vi "sub_NtripClient_TCP.vi"(8 "error in":errorcluster) -> (0 "error out":errorcluster)   [LabVIEW 2019]
uses:
  Ctrl/comm-ini-rw-close.ctl
  Ctrl/cmd_common.ctl
  Ctrl/cmd_RW.ctl
  Ctrl/cmd_ini-RW.ctl
panel:
  out "n":i32
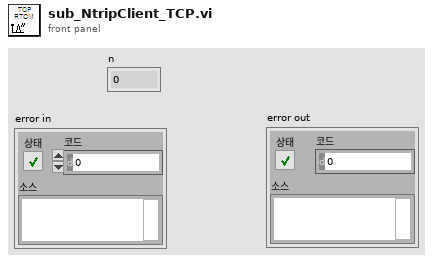
[diagram p1: front panel]
types:
  T1 = typedef "cmd_common.ctl" = enum16{"read", "write"}
  T2 = typedef "comm-ini-rw-close.ctl" = enum16{"ini", "write", "read", "close"}
  T3 = typedef "cmd_ini-RW.ctl" = enum16{"ini", "read", "write"}
  T4 = typedef "cmd_RW.ctl" = enum16{"read", "write"}
  T5 = typedef "GNSS-Ntrip config.ctl" = cluster{"Ntrip accounts DB":T6[], "Mount points":u16, "Ref r size":dbl, "TMarr limit":i32, "Sel NMEA type":enum16{"$GPGSV", "$GLGSV", "$GPGGA", "$GAGSV", "$GBGSV", "$GNGLL", "$GNGGA", "$GNGSA", "$GNRMC", "$GNVTG"}, "Local Time offset":u32, "GNSS Serial delay":u32, "Send Serial delay":u32, "Send Serial config":cluster{"NMEA out port":refnum<visa-resource-name>, "baud rate":u32}, "Mount point arr":string[], "Ntrip account DB index":u32}
  T6 = typedef "Ntrip_Account_db.ctl" = cluster{"address":string, "port ":u16, "id":string, "pwd":string, "ref pt":string}
  T7 = cluster{"Ntrip tcp":bool, "GNSS serial":bool, "RTCM serial":bool, "Send serial":bool}
  T8 = typedef "GNSS-Ntrip process val.ctl" = cluster{"GNSS time":string, "Ntrip conn":bool, "NMEA val":bool, "ycenter_TM":dbl, "xcenter_TM":dbl, "TM ref circles":cluster{"Y(E)":dbl, "X(N)":dbl}[], "RTCM recv-str":string, "GNSS Serail buff N":u32, "Sel NMEA type":enum16{"$GPGSV", "$GLGSV", "$GPGGA", "$GAGSV", "$GBGSV", "$GNGLL", "$GNGGA", "$GNGSA", "$GNRMC", "$GNVTG"}, "RTCM recv_sourcetable":string, "NMEA cluster":cluster{"GxGGA":string, "GxGSV":string, "GNRMC":string, "GxTXT":string, "GxGSA":string, "GxGLL":string}, "Sel NMEA str":string, "NMEA recv-str":string}
  T9 = typedef "GNSS-Ntrip ref.ctl" = cluster{"Mount point arr":refnum<vi>, "Select Mount points":refnum<vi>}
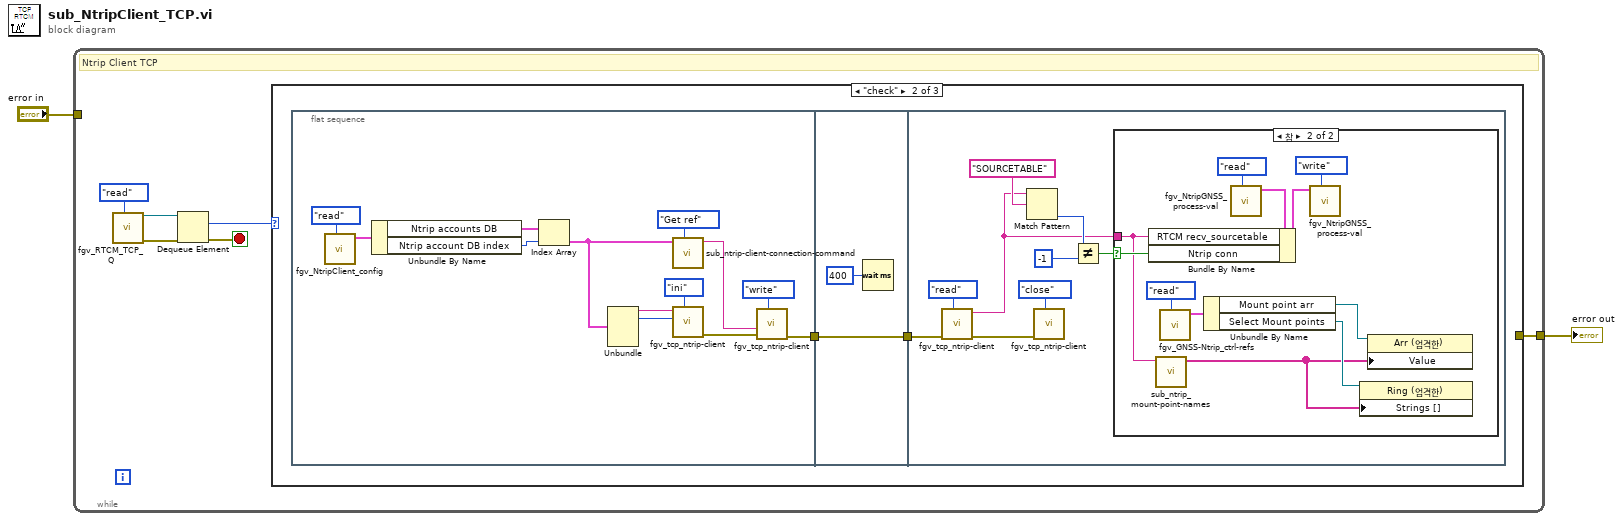
[diagram p0: block diagram]
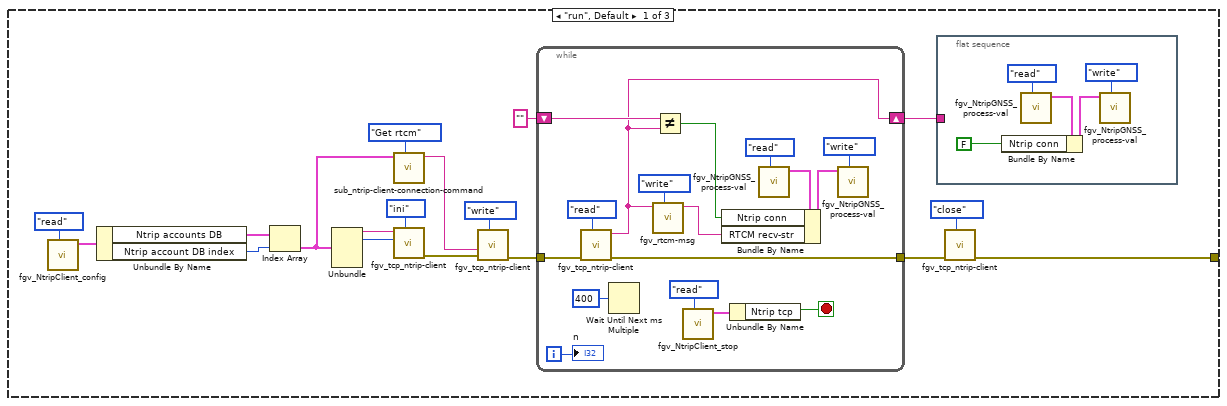
[diagram p2: hidden frame]
diagram:
  n1 = while {
    tunnel: "error in" -> [_]
    tunnel: [w3] -> w1
    stop <- w5 stop-if-true
    # "Ntrip Client TCP"
    n2 = call "fgv_RTCM_TCP_Q.vi"("cmd"=enum16{"create", "write", "read", "close"}."read") -> ("error out"=w7:errorcluster, "queue out"=w6:refnum<queue>)  [unwired: 9 in]
    n3 = Dequeue Element(queue=w6, error in (no error)=w7) -> (element=w4:enum16{"run", "check", "stop"}, error out=w5:errorcluster)  [unwired: 1 in, 2 out]
    n4 = case shown="\"check\"" w4 {
      tunnel: [w18 _ _] -> w3
      frame "run", Default {
        n5 = call "fgv_NtripClient_config.vi"("cmd"=cmd_common."read") -> ("config val out"=w16:T5)  [unwired: 10 in]
        n6 = Unbundle By Name(w16) -> ("Ntrip accounts DB"=w15:T6[], "Ntrip account DB index"=w9:u32)
        n7 = Index Array(array=w15, index=w9) -> (element=w14:T6)
        n8 = Unbundle(w14) -> ("address"=w13:string, "port"=w12:u16)  [unwired: 3 out]
        n9 = call "sub_ntrip-client-connection-command.vi"("cmd"=enum16{"Get ref", "Get rtcm"}."Get rtcm", "Current Ntrip account"=w14) -> ("hex"=w25:string)  [unwired: 9 in]
        n10 = call "fgv_tcp_ntrip-client.vi"("cmd"=comm-ini-rw-close."ini", "remote port"=w12, "address"=w13) -> ("error out"=w22:errorcluster)  [unwired: 7 in, 1 out]
        n11 = call "fgv_tcp_ntrip-client.vi"("cmd"=comm-ini-rw-close."write", "error in"=w22, "w-data"=w25) -> ("error out"=w21:errorcluster)  [unwired: 7 in, 1 out]
        n12 = while {
          tunnel: w21 -> [w43]
          tunnel: [w44] -> w19
          shift-right: [w33] -> w11
          shift-left: "" ("r-data") -> [w34]
          i -> [w35]
          stop <- w46 stop-if-true
          n13 = call "fgv_tcp_ntrip-client.vi"("cmd"=comm-ini-rw-close."read", "error in"=w43) -> ("error out"=w44:errorcluster, "r-data"=w33:string)  [unwired: 8 in]
          n14 = Wait Until Next ms Multiple(millisecond multiple=u32 400 ("ms 배수")) -> ()  [unwired: 1 out]
          n15 = call "fgv_rtcm-msg.vi"("cmd"=cmd_RW."write", "rtcm msg"=w33) -> ("rtcm msg out"=w36:string)  [unwired: 9 in]
          n16 = Not Equal?(x=w34, y=w33) -> (x != y?=w32:bool)
          n17 = call "fgv_NtripClient_stop.vi"("cmd"=cmd_ini-RW."read") -> ("local stops out"=w48:T7)  [unwired: 10 in]
          n18 = Unbundle By Name(w48) -> ("Ntrip tcp"=w46:bool)
          n19 = call "fgv_NtripGNSS_process-val.vi"("cmd"=cmd_ini-RW."read") -> ("process val out"=w37:T8)  [unwired: 10 in]
          n20 = Bundle By Name(cluster=w37, "Ntrip conn"=w32, "RTCM recv-str"=w36) -> (w38:T8)
          n21 = call "fgv_NtripGNSS_process-val.vi"("cmd"=cmd_ini-RW."write", "process val"=w38) -> ()  [unwired: 9 in, 1 out]
          "n" <- w35
        }
        n22 = flat-sequence {
          tunnel: w11 -> [_]
          frame #0 {
            n23 = call "fgv_NtripGNSS_process-val.vi"("cmd"=cmd_ini-RW."read") -> ("process val out"=w31:T8)  [unwired: 10 in]
            n24 = Bundle By Name(cluster=w31, "Ntrip conn"=FALSE) -> (w30:T8)
            n25 = call "fgv_NtripGNSS_process-val.vi"("cmd"=cmd_ini-RW."write", "process val"=w30) -> ()  [unwired: 9 in, 1 out]
          }
        }
        n26 = call "fgv_tcp_ntrip-client.vi"("cmd"=comm-ini-rw-close."close", "error in"=w19) -> ("error out"=w18:errorcluster)  [unwired: 8 in, 1 out]
      }
      frame "check" {
        n27 = flat-sequence {
          tunnel: [w58] -> w50
          tunnel: w50 -> [w65]
          tunnel: [w65] -> w49
          tunnel: w49 -> [w71]
          frame #0 {
            n28 = call "fgv_NtripClient_config.vi"("cmd"=cmd_common."read") -> ("config val out"=w57:T5)  [unwired: 10 in]
            n29 = Unbundle By Name(w57) -> ("Ntrip accounts DB"=w56:T6[], "Ntrip account DB index"=w51:u32)
            n30 = Index Array(array=w56, index=w51) -> (element=w54:T6)
            n31 = Unbundle(w54) -> ("address"=w53:string, "port"=w52:u16)  [unwired: 3 out]
            n32 = call "sub_ntrip-client-connection-command.vi"("cmd"=enum16{"Get ref", "Get rtcm"}."Get ref", "Current Ntrip account"=w54) -> ("hex"=w63:string)  [unwired: 9 in]
            n33 = call "fgv_tcp_ntrip-client.vi"("cmd"=comm-ini-rw-close."ini", "remote port"=w52, "address"=w53) -> ("error out"=w59:errorcluster)  [unwired: 7 in, 1 out]
            n34 = call "fgv_tcp_ntrip-client.vi"("cmd"=comm-ini-rw-close."write", "error in"=w59, "w-data"=w63) -> ("error out"=w58:errorcluster)  [unwired: 7 in, 1 out]
          }
          frame #1 {
            n35 = Wait (ms)(milliseconds to wait=u32 400 ("ms 배수")) -> ()  [unwired: 1 out]
          }
          frame #2 {
            n36 = call "fgv_tcp_ntrip-client.vi"("cmd"=comm-ini-rw-close."read", "error in"=w71) -> ("error out"=w74:errorcluster, "r-data"=w66:string)  [unwired: 8 in]
            n37 = Match Pattern(string=w66, regular expression="SOURCETABLE" ("정규식")) -> (offset past match=w70:i32)  [unwired: 1 in, 3 out]
            n38 = call "fgv_tcp_ntrip-client.vi"("cmd"=comm-ini-rw-close."close", "error in"=w74) -> ()  [unwired: 8 in, 2 out]
            n39 = Not Equal?(x=w70, y=-1) -> (x != y?=w67:bool)
            n40 = case shown="참" w67 {
              selector: w67 -> [_ w81]
              tunnel: w66 -> [_ w80]
              frame False {
              }
              frame True {
                n41 = call "sub_ntrip_mount-point-names.vi"("ntrip str"=w80) -> ("mount points"=w75:string[])  [unwired: 10 in]
                n42 = call "fgv_GNSS-Ntrip_ctrl-refs.vi"("cmd"=cmd_common."read") -> ("ref 2"=w78:T9)  [unwired: 10 in]
                n43 = Unbundle By Name(w78) -> ("Mount point arr"=w77:refnum<vi>, "Select Mount points"=w76:refnum<vi>)
                n44 = call "fgv_NtripGNSS_process-val.vi"("cmd"=cmd_ini-RW."read") -> ("process val out"=w82:T8)  [unwired: 10 in]
                n45 = Bundle By Name(cluster=w82, "RTCM recv_sourcetable"=w80, "Ntrip conn"=w81) -> (w83:T8)
                n46 = call "fgv_NtripGNSS_process-val.vi"("cmd"=cmd_ini-RW."write", "process val"=w83) -> ()  [unwired: 9 in, 1 out]
                n47 = property on="프로퍼티 노드" class="Ring (엄격한)"(reference=w76, "Strings []"=w75) -> ()  [unwired: 1 in, 2 out]
                n48 = property on="프로퍼티 노드" class="Arr (엄격한)"(reference=w77, "Value"=w75) -> ()  [unwired: 1 in, 2 out]
              }
            }
          }
        }
      }
      frame "stop" {
      }
    }
  }
  "error out" <- w1
